vi "Lint VI.vi"(8 "Error In":errorcluster, 10 "Results In":T1[](array[typedef]), 11 "Project Item In":refnum<vi>) -> (0 "Error Out":errorcluster, 2 "Results Out":T1[](array[typedef]), 3 "Project Item Out":refnum<vi>)   [LabVIEW 2018, in "Scripts.lvlib"]
uses:
  Scripts.lvlib
  Project Item Lint Result.ctl
  VI Control Lint Result.ctl
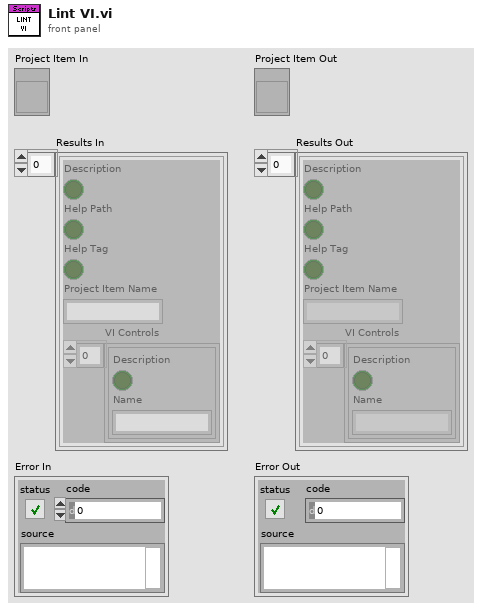
[diagram p1: front panel]
types:
  T1 = typedef "Scripts.lvlib/Project Item Lint Result.ctl" = cluster{"Description":bool, "Help Path":bool, "Help Tag":bool, "Project Item Name":string, "VI Controls":T2[]}
  T2 = typedef "Scripts.lvlib/VI Control Lint Result.ctl" = cluster{"Description":bool, "Name":string}
  T3 = enum32{"invalid scope", "public", "private", "protected", "community"}
  T4 = enum32{"invalid VI type", "Standard VI", "Control VI", "Global VI", "Polymorphic VI", "Configuration VI", "SubSystem", "Facade VI", "Method VI", "Statechart Diagram VI"}
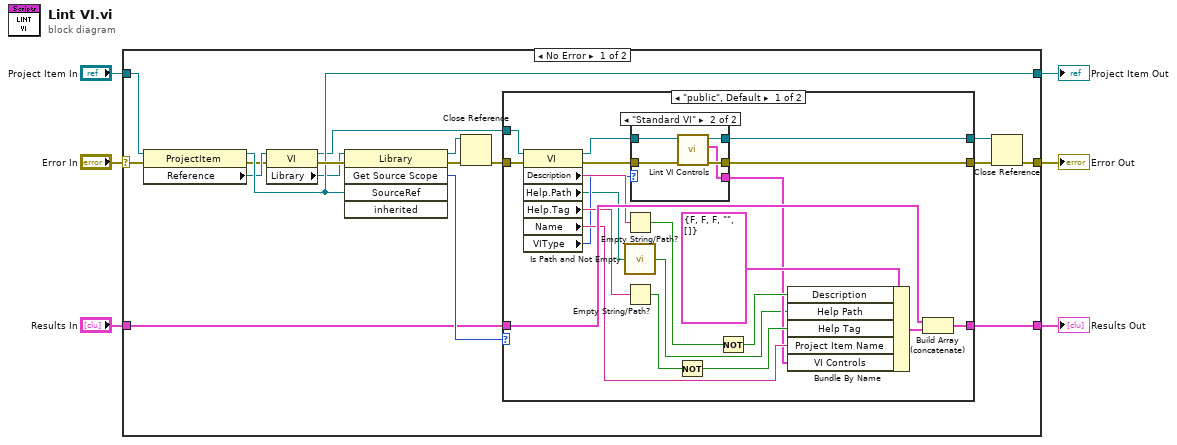
[diagram p0: block diagram]
diagram:
  n1 = case shown="No Error" "Error In" {
    selector: "Error In" -> [w7 w56]
    tunnel: [w18 w57] -> w6
    tunnel: [w11 w55] -> w5
    tunnel: "Results In" -> [w10 w55]
    tunnel: [w9 w56] -> w3
    tunnel: "Project Item In" -> [w8 w57]
    frame No Error {
      n2 = property class="ProjectItem"(reference=w8, error in=w7) -> (reference out=w18:refnum<vi>, error out=w12:errorcluster, "Reference"=w15:refnum<vi>)
      n3 = property class="VI"(reference=w15, error in=w12) -> (reference out=w16:refnum<vi>, error out=w19:errorcluster, "Library"=w17:refnum<vi>)
      n4 = invoke class="Library" method="Get Source Scope"(reference=w17, error in=w19, "SourceRef"=w18) -> (reference out=w20:refnum<vi>, error out=w21:errorcluster, "GetSourceScope"=w23:T3)  [unwired: 2 in, 2 out]
      n5 = Close Reference(reference=w20, error in (no error)=w21) -> (error out=w22:errorcluster)
      n6 = case shown="\"public\", Default" w23 {
        tunnel: w10 -> [w44 w54]
        tunnel: [w43 w54] -> w11
        tunnel: [w33 w53] -> w13
        tunnel: [w32 w52] -> w14
        tunnel: w16 -> [w27 w53]
        tunnel: w22 -> [w26 w52]
        frame "public", Default {
          n7 = property class="VI"(reference=w27, error in=w26) -> (reference out=w34:refnum<vi>, error out=w31:errorcluster, "Description"=w41:string, "Help.Path"=w25:path, "Help.Tag"=w40:string, "Name"=w39:string, "VIType"=w28:T4)
          n8 = Empty String/Path?(string/path=w41) -> (empty?=w38:bool)
          n9 = call <vilib>:"Is Path and Not Empty.vi"("path"=w25) -> ("Is Path and Not Empty?"=w24:bool)  [unwired: 4 in]
          n10 = Empty String/Path?(string/path=w40) -> (empty?=w37:bool)
          n11 = case shown="\"Standard VI\"" w28 {
            tunnel: w34 -> [w46 w51]
            tunnel: [w46 w50] -> w33
            tunnel: [w45 w49] -> w32
            tunnel: w31 -> [w45 w48]
            tunnel: [_ w47] -> w30
            frame "invalid VI type", Default {
            }
            frame "Standard VI" {
              n12 = call "Lint VI Controls.vi"("Error In"=w48, "VI In"=w51) -> ("Error Out"=w49:errorcluster, "Results"=w47:T2[], "VI Out"=w50:refnum<vi>)  [unwired: 7 in]
            }
          }
          n13 = Not(x=w37) -> (.not. x?=w35:bool)
          n14 = Not(x=w38) -> (.not. x?=w36:bool)
          n15 = Bundle By Name(cluster=T1 {"Description"=FALSE, "Help Path"=FALSE, "Help Tag"=FALSE, "Project Item Name"="", "VI Controls"=[]} ("Lint Result"), "Description"=w36, "Help Path"=w24, "Help Tag"=w35, "Project Item Name"=w39, "VI Controls"=w30) -> (w29:T1)
          n16 = Build Array (concatenate)(w44, w29) -> (w43:T1[])
        }
        frame "private" {
        }
      }
      n17 = Close Reference(reference=w13, error in (no error)=w14) -> (error out=w9:errorcluster)
    }
    frame Error {
    }
  }
  "Project Item Out" <- w6
  "Results Out" <- w5
  "Error Out" <- w3
